vi "PID Process.vi"(0 "PID gains":T3={"proportional gain (Kc)"=1.0, "integral time (Ti, min)"=0.01, "derivative time (Td, min)"=0.0} {"derivative time (Td, min)" format="%.12f"; "integral time (Ti, min)" format="%.12f"; "proportional gain (Kc)" format="%.12f"}, 1 "Dy Value":T2 {"Wout" format="%.2f"; "Torque Value" format="%.2f"}, 5 "Set Value":dbl, 7 "process variable":dbl format="%.2f", 9 "Read Unit":T1(ring)=enum."oz.ft" caption="扭力輸出單位", 11 "PID Mode":enum16{"Torque", "Power"}(ring), 12 "reinitialize? (F)":bool) -> (4 "Torque Value Out":dbl min=0.0 max=100.0 step=0.1)   [LabVIEW 2024]
uses:
  <vilib>/addons/control/pid/pid.llb/PID (DBL).vi
  <vilib>/addons/control/pid/NI_PID_pid.lvlib
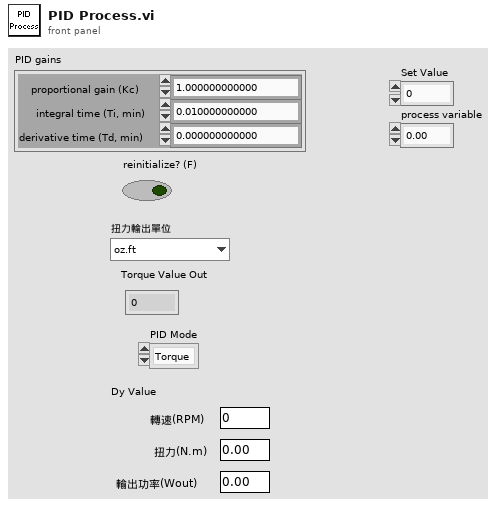
[diagram p1: front panel]
types:
  T1 = enum16{"oz.in", "oz.ft", "lb.in", "lb.ft", "g.cm", "Kg.cm", "mN.m", "cN.m", "N.m"}
  T2 = cluster{"Speed Value":dbl, "Torque Value":dbl, "Wout":dbl}
  T3 = cluster{"proportional gain (Kc)":dbl, "integral time (Ti, min)":dbl, "derivative time (Td, min)":dbl}
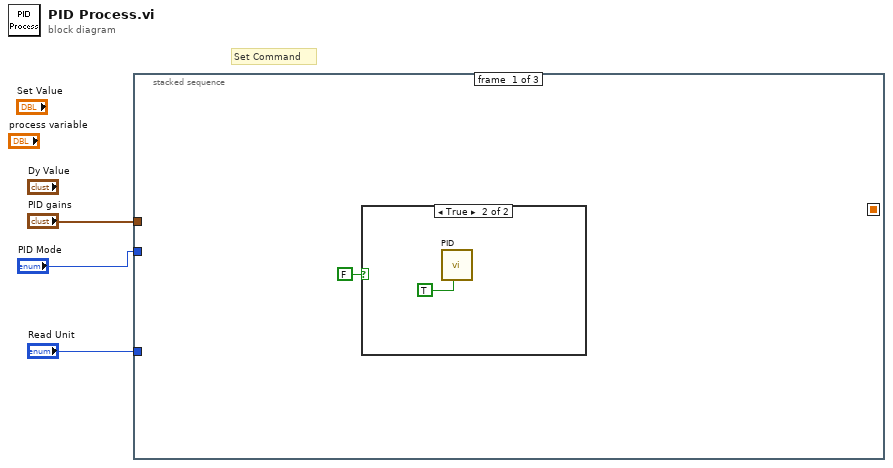
[diagram p0: block diagram]
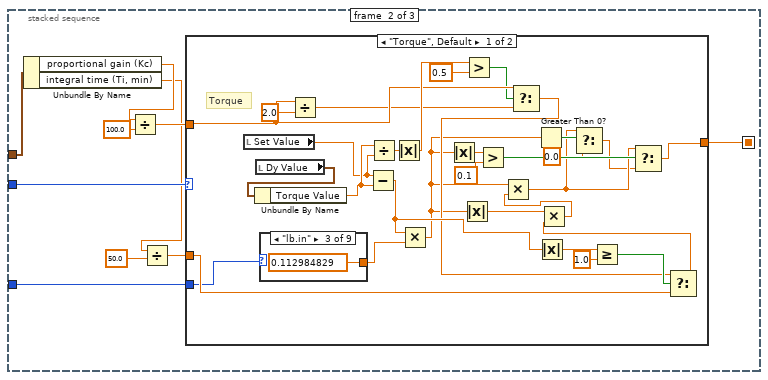
[diagram p3: hidden frame]
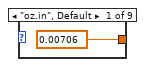
[diagram p4: hidden frame]
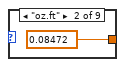
[diagram p5: hidden frame]
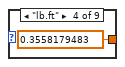
[diagram p6: hidden frame]
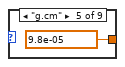
[diagram p7: hidden frame]
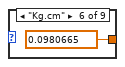
[diagram p8: hidden frame]
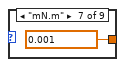
[diagram p9: hidden frame]
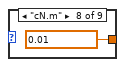
[diagram p10: hidden frame]
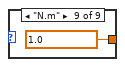
[diagram p11: hidden frame]
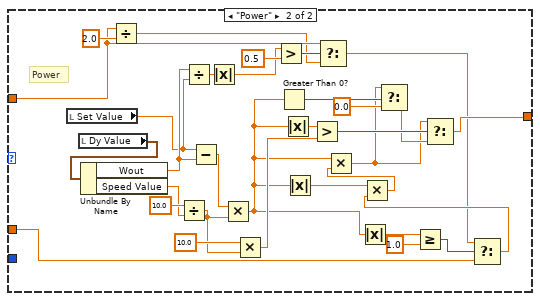
[diagram p12: hidden frame]
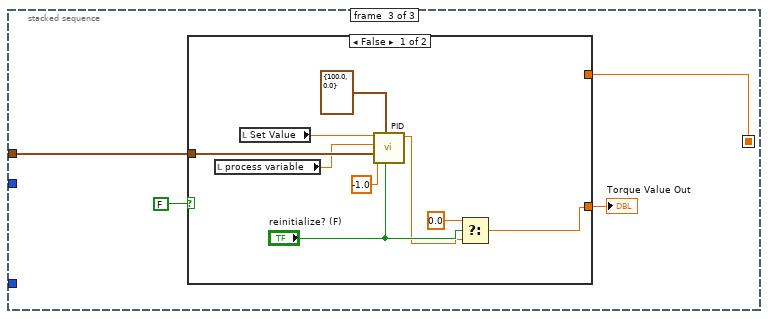
[diagram p13: hidden frame]
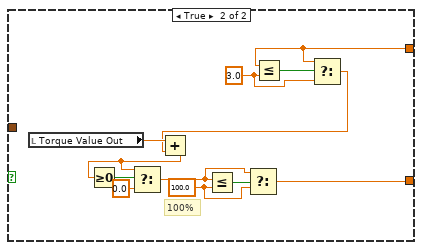
[diagram p14: hidden frame]
diagram:
  # "Set Command"
  n1 = stacked-sequence {
    seq-local: [_ w14 _] -> [_ _ w90]
    tunnel: "PID Mode" -> [_ w15 _]
    tunnel: "Read Unit" -> [_ w9 _]
    tunnel: "PID gains" -> [_ w8 w88]
    frame #0 {
      n2 = case shown="True" FALSE {
        frame False {
        }
        frame True {
          n3 = call-poly <vilib>:"PID.vi"("reinitialize? (F)"=TRUE) -> ()  [unwired: 9 in, 2 out]
        }
      }
    }
    frame #1 {
      n4 = Unbundle By Name(w8) -> ("proportional gain (Kc)"=w7:dbl, "integral time (Ti, min)"=w6:dbl)
      n5 = Divide(x=w7, y=100.0) -> (x/y=w12:dbl)
      n6 = Divide(x=w6, y=50.0) -> (x/y=w10:dbl)
      n7 = case shown="\"Torque\", Default" w15 {
        tunnel: [w34 w74] -> w14
        tunnel: w12 -> [w28 w66]
        tunnel: w10 -> [w35 w75]
        tunnel: w9 -> [w17 _]
        frame "Torque", Default {
          # "Torque"
          n8 = local read "Set Value"() -> (w24:dbl)
          n9 = local read "Dy Value"() -> (w45:T2)
          n10 = Unbundle By Name(w45) -> ("Torque Value"=w25:dbl)
          n11 = case shown="\"lb.in\"" w17 {
            tunnel: [0.00706 0.08472 0.112984829 0.3558179483 9.8e-05 0.0980665 0.001 0.01 1.0] -> w16
            frame "oz.in", Default {
            }
            frame "oz.ft" {
            }
            frame "lb.in" {
            }
            frame "lb.ft" {
            }
            frame "g.cm" {
            }
            frame "Kg.cm" {
            }
            frame "mN.m" {
            }
            frame "cN.m" {
            }
            frame "N.m" {
            }
          }
          n12 = Divide(x=w28, y=2.0) -> (x/y=w27:dbl)
          n13 = Subtract(x=w24, y=w25) -> (x-y=w40:dbl)
          n14 = Divide(x=w25, y=w24) -> (x/y=w33:dbl)
          n15 = Absolute Value(x=w33) -> (abs(x)=w31:dbl)
          n16 = Multiply(x=w40, y=w16) -> (x*y=w22:dbl)
          n17 = Absolute Value(x=w22) -> (abs(x)=w41:dbl)
          n18 = Absolute Value(x=w22) -> (abs(x)=w43:dbl)
          n19 = Greater?(x=w31, y=0.5) -> (0:w26:bool)
          n20 = Greater?(x=w41, y=0.1) -> (0:w23:bool)
          n21 = Select(t=w28, s=w26, f=w27) -> (s? t:f=w32:dbl)
          n22 = Greater Than 0?(x=w22) -> (x > 0?=w21:bool)
          n23 = Absolute Value(x=w40) -> (abs(x)=w39:dbl)
          n24 = Greater Or Equal?(x=w39, y=1.0) -> (x >= y?=w37:bool)
          n25 = Select(t=w32, s=w37, f=w35) -> (s? t:f=w36:dbl)
          n26 = Multiply(x=w43, y=w36) -> (x*y=w44:dbl)
          n27 = Multiply(x=w22, y=w44) -> (x*y=w20:dbl)
          n28 = Select(t=w20, s=w21, f=0.0) -> (s? t:f=w19:dbl)
          n29 = Select(t=w20, s=w23, f=w19) -> (s? t:f=w34:dbl)
        }
        frame "Power" {
          # "Power"
          n30 = local read "Set Value"() -> (w71:dbl)
          n31 = local read "Dy Value"() -> (w86:T2)
          n32 = Unbundle By Name(w86) -> ("Wout"=w72:dbl, "Speed Value"=w62:dbl)
          n33 = Divide(x=w66, y=2.0) -> (x/y=w65:dbl)
          n34 = Divide(x=10.0 ("y"), y=w62) -> (x/y=w64:dbl)
          n35 = Divide(x=w72, y=w71) -> (x/y=w73:dbl)
          n36 = Subtract(x=w71, y=w72) -> (x-y=w81:dbl)
          n37 = Absolute Value(x=w73) -> (abs(x)=w68:dbl)
          n38 = Multiply(x=w81, y=w64) -> (x*y=w55:dbl)
          n39 = Multiply(x=10.0 ("y"), y=w64) -> (x*y=w76:dbl)
          n40 = Greater?(x=w68, y=0.5) -> (0:w70:bool)
          n41 = Greater Than 0?(x=w55) -> (x > 0?=w60:bool)
          n42 = Absolute Value(x=w55) -> (abs(x)=w82:dbl)
          n43 = Absolute Value(x=w55) -> (abs(x)=w84:dbl)
          n44 = Greater?(x=w82, y=w76) -> (0:w83:bool)
          n45 = Select(t=w66, s=w70, f=w65) -> (s? t:f=w61:dbl)
          n46 = Absolute Value(x=w55) -> (abs(x)=w80:dbl)
          n47 = Greater Or Equal?(x=w80, y=1.0) -> (x >= y?=w79:bool)
          n48 = Select(t=w61, s=w79, f=w75) -> (s? t:f=w78:dbl)
          n49 = Multiply(x=w84, y=w78) -> (x*y=w85:dbl)
          n50 = Multiply(x=w55, y=w85) -> (x*y=w57:dbl)
          n51 = Select(t=w57, s=w60, f=0.0) -> (s? t:f=w58:dbl)
          n52 = Select(t=w57, s=w83, f=w58) -> (s? t:f=w74:dbl)
        }
      }
    }
    frame #2 {
      n53 = case shown="False" FALSE ("PID Select") {
        tunnel: [w92 w106] -> w87
        tunnel: w90 -> [_ w101]
        tunnel: w88 -> [w98 _]
        frame False {
          n54 = local read "process variable"() -> (w95:dbl)
          n55 = local read "Set Value"() -> (w96:dbl)
          n56 = call-poly <vilib>:"PID.vi"("reinitialize? (F)"="reinitialize? (F)", "output range"=cluster{"output high":dbl, "output low":dbl} {"output high"=100.0, "output low"=0.0}, "dt (s)"=-1.0, "PID gains"=w98, "process variable"=w95, "setpoint"=w96) -> ("output"=w91:dbl)  [unwired: 4 in, 1 out]
          n57 = Select(t=0.0, s="reinitialize? (F)", f=w91) -> (s? t:f=w92:dbl)
        }
        frame True {
          w100 = 3.0 ("y")
          w107 = 100.0 ("y")
          # "100%"
          n58 = local read "Torque Value Out"() -> (w105:dbl)
          n59 = Less Or Equal?(x=w101, y=w100) -> (x <= y?=w103:bool)
          n60 = Select(t=w101, s=w103, f=w100) -> (s? t:f=w102:dbl)
          n61 = Add(x=w105, y=w102) -> (x+y=w104:dbl)
          n62 = Greater Or Equal To 0?(x=w104) -> (x >= 0?=w111:bool)
          n63 = Select(t=w104, s=w111, f=0.0) -> (s? t:f=w108:dbl)
          n64 = Less Or Equal?(x=w108, y=w107) -> (x <= y?=w109:bool)
          n65 = Select(t=w108, s=w109, f=w107) -> (s? t:f=w106:dbl)
        }
      }
      "Torque Value Out" <- w87
    }
  }
